vi "Configure Frequency.vi"(8 "error in (no error)":errorcluster, 10 "Frequency [Hz]":dbl, 11 "SigGen-SMBV in":refnum<class "SigGen-SMBV.lvclass">) -> (0 "error out":errorcluster, 3 "SigGen-SMBV out":refnum<class "SigGen-SMBV.lvclass">)   [LabVIEW 2020, in "SigGen-SMBV.lvclass"]
uses:
  SigGen-SMBV.lvclass
  C:/Sandbox/Git_Sandbox/WiSpry Test Framework source code (LV20)/WiSpry Test Framework/Instruments/Signal Generator/Signal Generator.lvclass
  C:/Sandbox/Git_Sandbox/WiSpry Test Framework source code (LV20)/WiSpry Test Framework/Instruments/Instrument.lvclass
  Signal Generator.lvclass/Signal Generator.ctl
  Instrument.lvclass/Instrument.ctl
  Signal Generator.lvclass
  Instrument.lvclass
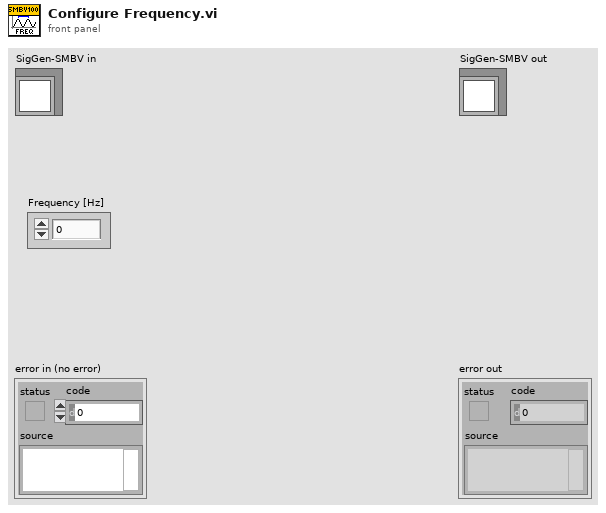
[diagram p1: front panel]
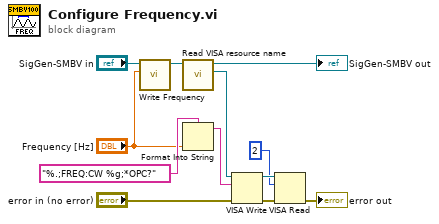
[diagram p0: block diagram]
diagram:
  n1 = call "Write Frequency.vi"("Frequency"="Frequency [Hz]", "Signal Generator in"="SigGen-SMBV in") -> ("Signal Generator out"=w11:refnum<class "SigGen-SMBV.lvclass">)  [unwired: 9 in]
  n2 = call "Read VISA resource name.vi"("Instrument in"=w11) -> ("VISA resource name"=w7:refnum<visa-resource-name>, "Instrument out"=→"SigGen-SMBV out":refnum<class "SigGen-SMBV.lvclass">)  [unwired: 9 in]
  n3 = Format Into String(format string="%.;FREQ:CW %g;*OPC?", "Frequency [Hz]") -> (resulting string=w6:string)  [unwired: 2 in, 1 out]
  n4 = VISA Write(VISA resource name=w7, write buffer=w6, error in (no error)="error in (no error)") -> (VISA resource name out=w3:refnum<visa-resource-name>, error out=w4:errorcluster)  [unwired: 1 out]
  n5 = VISA Read(VISA resource name=w3, byte count=u32 2, error in (no error)=w4) -> (error out=→"error out":errorcluster)  [unwired: 3 out]
